vi "ChartSettings2.vi"(1 "Numeric":dbl format="%#_13g", 2 "XY Graph Ref in":refnum<vi>) -> ()   [LabVIEW 2013]
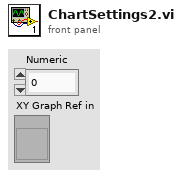
[diagram p1: front panel]
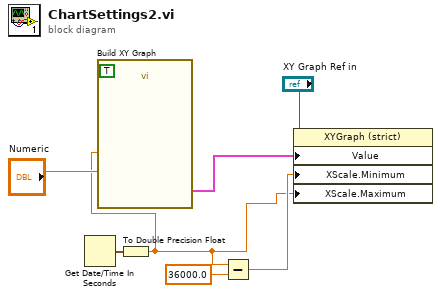
[diagram p0: block diagram]
diagram:
  n1 = Get Date/Time In Seconds() -> (seconds since 1Jan1904=w7:timestamp)
  n2 = To Double Precision Float(number=w7) -> (double precision float=w1:dbl)
  n3 = call "Build XY Graph"("Enable"=TRUE, "Y Input"="Numeric", "X Input"=w1) -> ("XY Graph"=w2:cluster{"X":dbl[], "Y":dbl[]}[])  [unwired: 7 in, 1 out]
  n4 = Subtract(x=w1, y=36000.0) -> (x-y=w3:dbl)
  n5 = property on="Property Node" class="XYGraph (strict)"(reference="XY Graph Ref in", "Value"=w2, "XScale.Minimum"=w3, "XScale.Maximum"=w1) -> ()  [unwired: 1 in, 2 out]
